vi "加速度_峭度指标.vi"(10 "均方根值":dbl format="%0.2p", 11 "信号X":dbl[](array[numeric])) -> (3 "峭度指标":dbl)   [LabVIEW 2014]
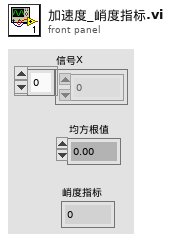
[diagram p1: front panel]
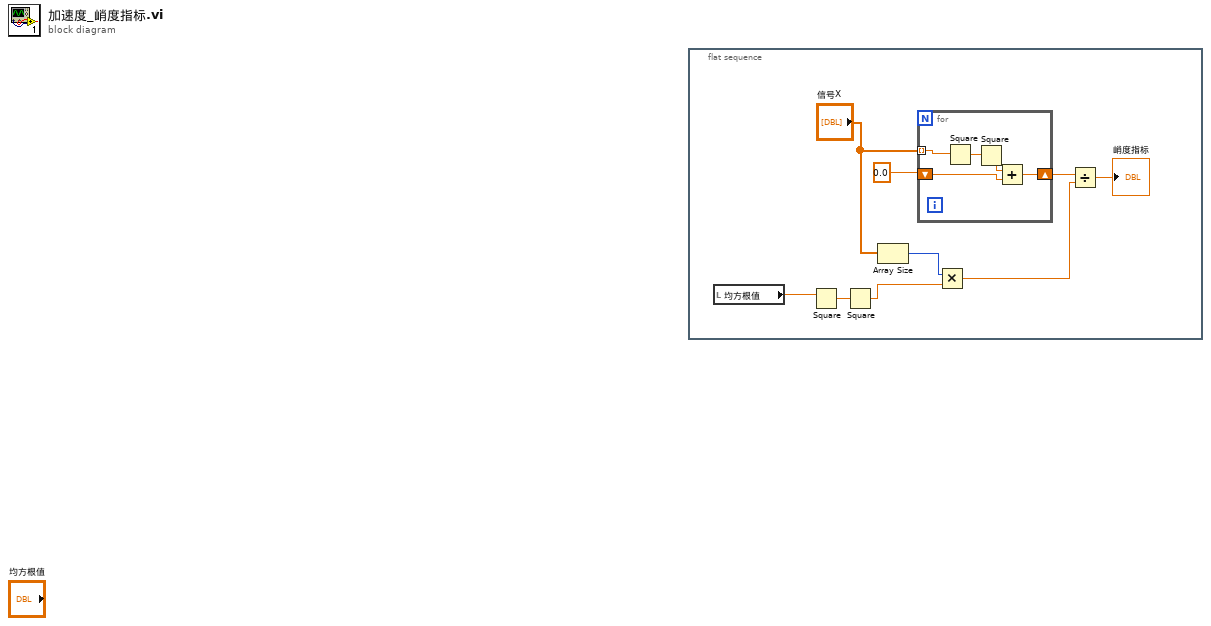
[diagram p0: block diagram]
diagram:
  n1 = flat-sequence {
    frame #0 {
      n2 = local read "均方根值"() -> (w4:dbl)
      n3 = Square(x=w4) -> (x^2=w3:dbl)
      n4 = Square(x=w3) -> (x^2=w2:dbl)
      n5 = Array Size(array="信号X") -> (size(s)=w6:i32)
      n6 = for {
        tunnel: "信号X" -> [w14] mode=indexing
        shift-right: [w10] -> w8
        shift-left: 0.0 -> [w11]
        n7 = Square(x=w14) -> (x^2=w13:dbl)
        n8 = Square(x=w13) -> (x^2=w12:dbl)
        n9 = Add(x=w12, y=w11) -> (x+y=w10:dbl)
      }
      n10 = Multiply(x=w6, y=w2) -> (x*y=w5:dbl)
      n11 = Divide(x=w8, y=w5) -> (x/y=→"峭度指标":dbl)
    }
  }
